vi "Recall aNETka (batch).vi"() -> ()   [LabVIEW 2010]
uses:
  <vilib>/Utility/file.llb/Read From Spreadsheet File (DBL).vi
panel:
  in  "Case Constant\n(See Context Help) 2":bool
  in  "Case Constant\n(See Context Help)":bool
  out "Output Array":sgl[](array[numeric])=[0.04986743, 0.15020862, 0.24986751, 0.34442046, 0.44537312, 0.54999864, 0.6508218, 0.7484142, 0.8519573, 0.94851804] format="%.2f"
  out "New file:":path=path "D:/aNETka/example 2 inputs, 1 output (aNETka).txt"
  out "Waveform Graph":sgl[][](graph)=[[0.04986743], [0.15020862], [0.24986751], [0.34442046], [0.44537312], [0.54999864], [0.6508218], [0.7484142], [0.8519573], [0.94851804]]
  out "aNETka config":i32[](array[numeric])=[2, 5, 1]
  out "Input file:":path=path "D:/aNETka/example 2 inputs, 1 output.txt"
  out "Function":enum16{"Linear", "Sigmoid", "Tangent hyp."}(ring)=enum."Sigmoid"
  out "aNETka config":i32[](array[numeric])=[2, 5, 1] min=0 max=100 step=1
  out "aNETka configuration":cluster{dbl[], dbl[]}[](graph)=[{[2.0, 3.0], [5.5, 3.5]}, {[2.0, 3.0], [4.5, 3.5]}, {[2.0, 3.0], [3.5, 3.5]}, {[2.0, 3.0], [2.5, 3.5]}, {[2.0, 3.0], [1.5, 3.5]}, {[1.0, 2.0], [4.0, 1.5]}, {[1.0, 2.0], [4.0, 2.5]}, {[1.0, 2.0], [4.0, 3.5]}, {[1.0, 2.0], [4.0, 4.5]}, {[1.0, 2.0], [4.0, 5.5]}, {[1.0, 2.0], [3.0, 1.5]}, {[1.0, 2.0], [3.0, 2.5]}, {[1.0, 2.0], [3.0, 3.5]}, {[1.0, 2.0], [3.0, 4.5]}, {[1.0, 2.0], [3.0, 5.5]}]
  # "Inputs"
  # "Outputs"
  # "(Hidden layers)"
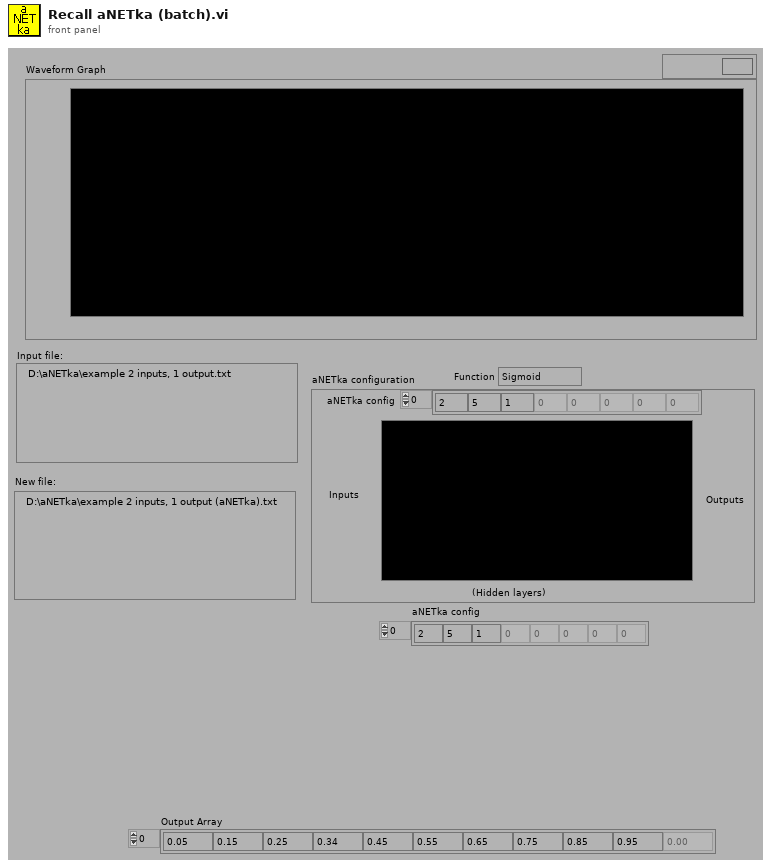
[diagram p1: front panel]
types:
  T1 = enum32{"existing file", "new file", "new or existing file", "existing dir", "new dir", "new or existing dir", "existing file (use LLBs)", "new file (use LLBs)", "new or existing file (use LLBs)", "new or existing file or directory (use LLBs)"}
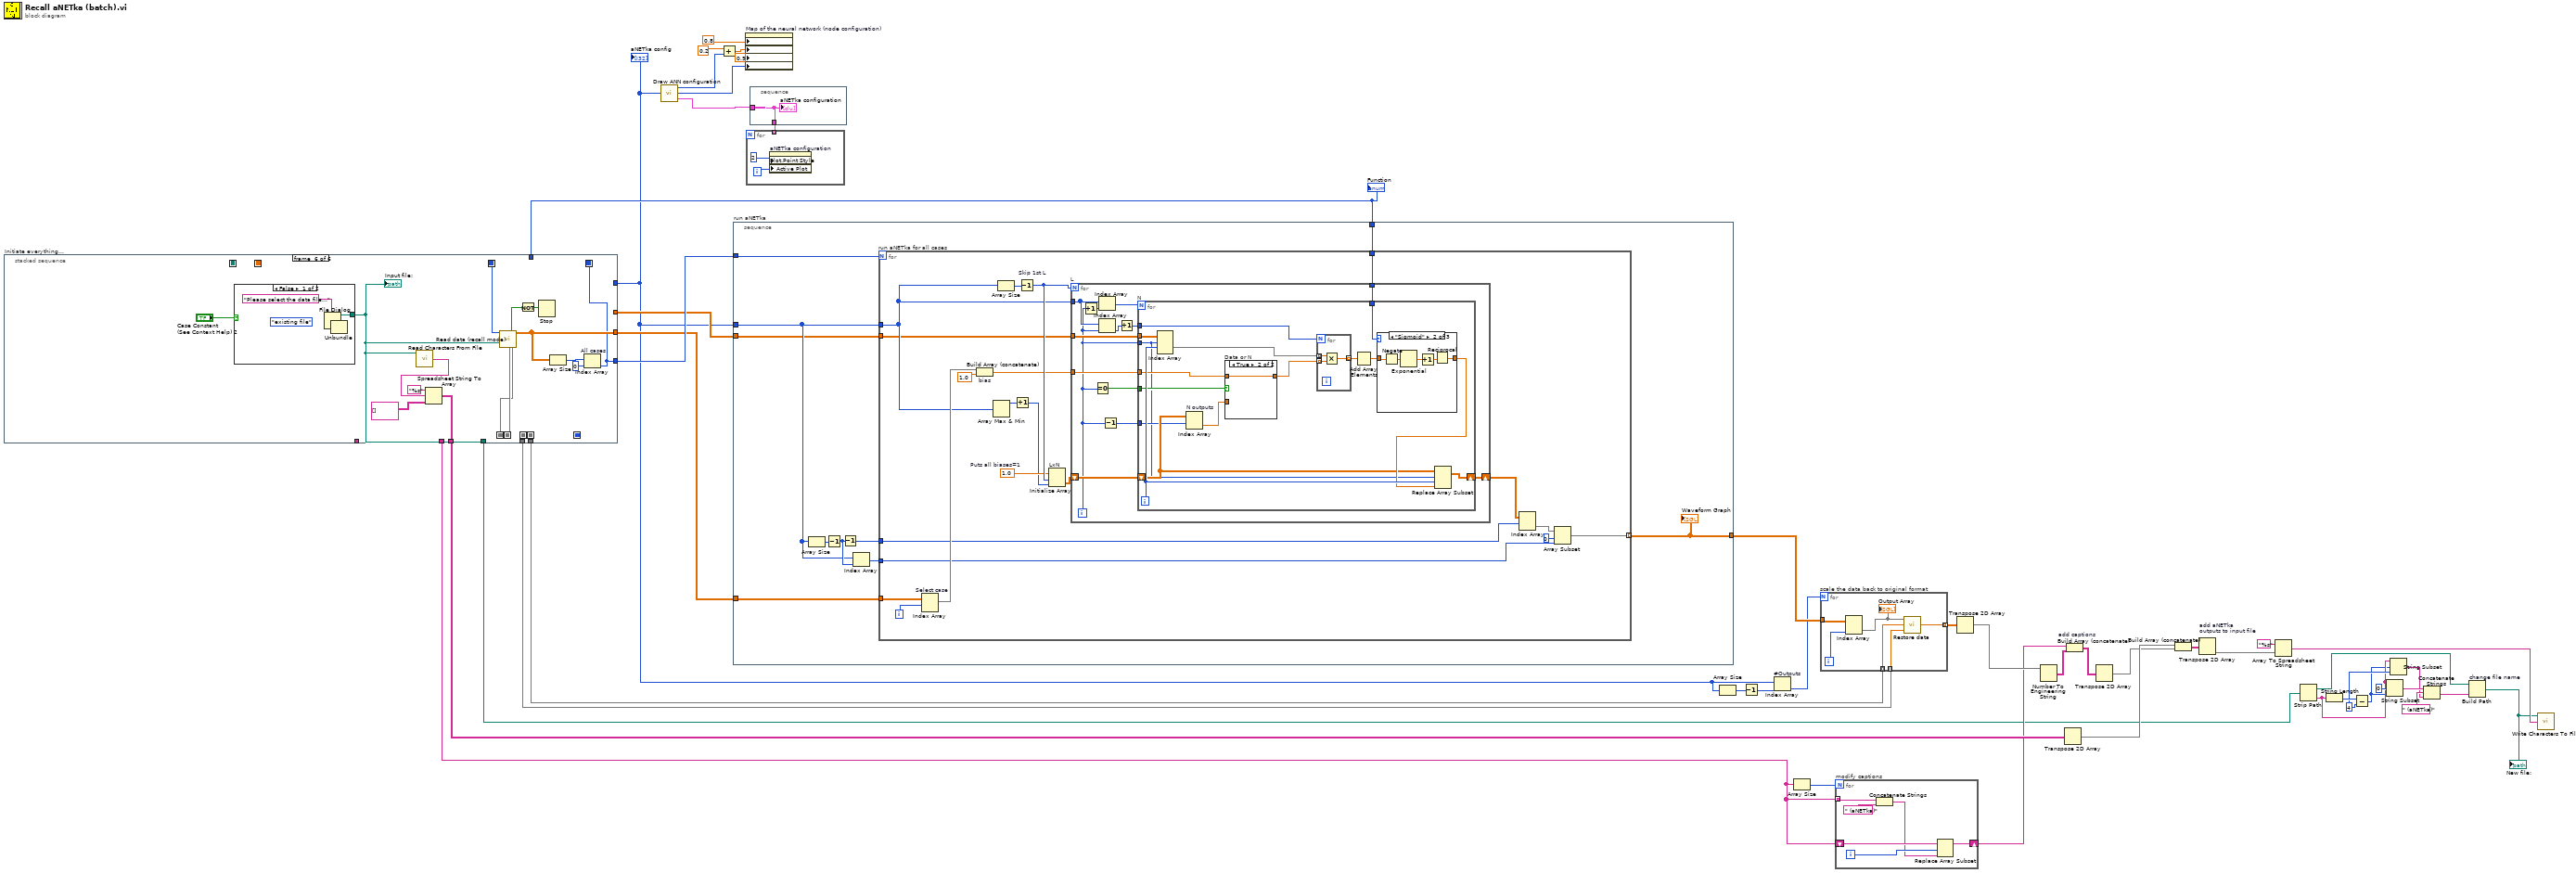
[diagram p0: block diagram]
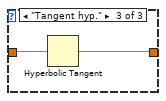
[diagram p3: hidden frame]
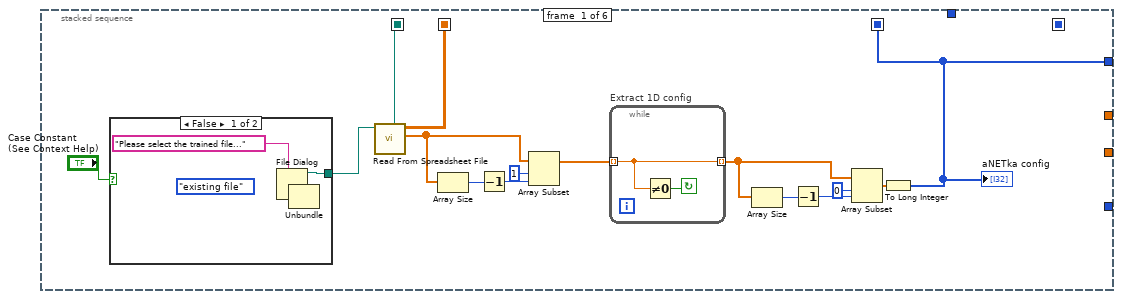
[diagram p5: hidden frame]
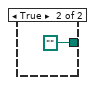
[diagram p6: hidden frame]
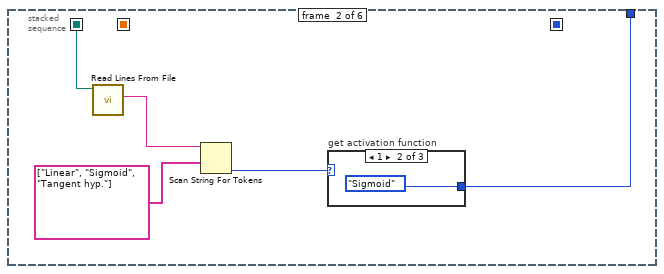
[diagram p7: hidden frame]
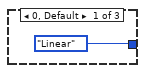
[diagram p8: hidden frame]
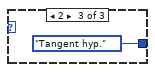
[diagram p9: hidden frame]
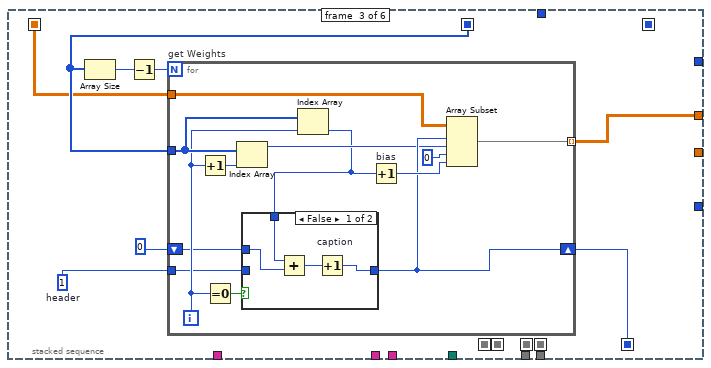
[diagram p10: hidden frame]
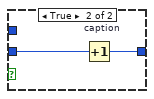
[diagram p11: hidden frame]
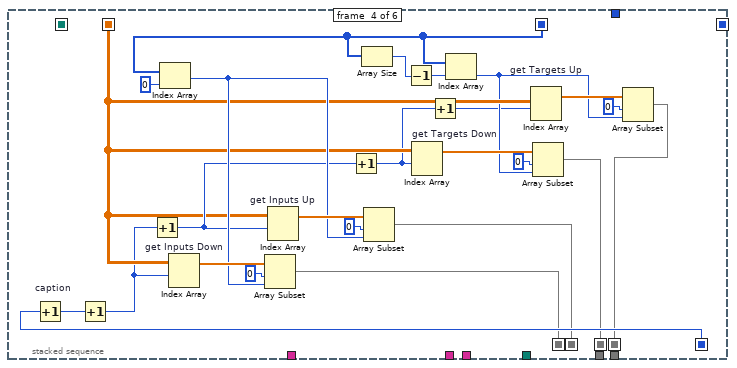
[diagram p12: hidden frame]
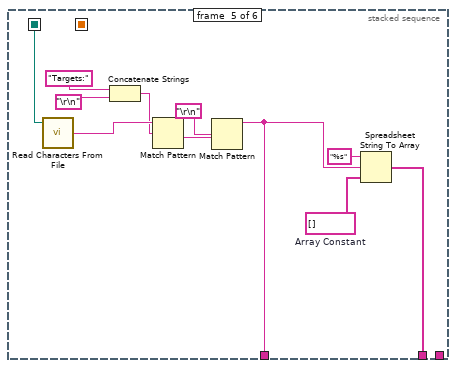
[diagram p13: hidden frame]
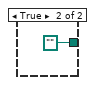
[diagram p14: hidden frame]
diagram:
  w11 = 4 ("y")
  n1 = stacked-sequence "Initiate everything..." {
    seq-local: [w49 _ _ _ _ _] -> [_ _ w80 w115 _ w150]
    seq-local: [_ _ _ _ _ w146] -> [_ _ _ _ _ _]
    seq-local: [w50 _ _ _ _ _] -> [_ _ w79 w110 _ _]
    seq-local: [w48 _ _ _ _ _] -> [_ w71 _ _ w137 _]
    seq-local: [_ _ w75 _ _ _] -> [_ _ _ w126 _ _]
    seq-local: [_ _ _ w105 _ _] -> [_ _ _ _ _ w143]
    seq-local: [_ _ _ w104 _ _] -> [_ _ _ _ _ w144]
    seq-local: [_ _ _ w102 _ _] -> [_ _ _ _ _ _]
    seq-local: [_ _ _ w103 _ _] -> [_ _ _ _ _ _]
    tunnel: [w49 _ _ _ _ _] -> w28
    tunnel: [_ w67 _ _ _ _] -> w37
    tunnel: [_ _ _ _ _ w147] -> w34
    tunnel: [_ _ _ _ _ w146] -> w36
    tunnel: [_ _ _ _ _ w138] -> w2
    tunnel: [_ _ w76 _ _ _] -> w35
    tunnel: [_ _ _ _ w130 _] -> _
    tunnel: [_ _ _ w103 _ _] -> w27
    tunnel: [_ _ _ w102 _ _] -> w26
    tunnel: [_ _ _ _ _ w139] -> w25
    tunnel: [_ _ _ _ w127 _] -> w17
    frame #0 {
      n2 = case shown="False" "Case Constant\n(See Context Help)" {
        tunnel: [w64 path ""] -> w46
        frame False {
          (unwired) T1."existing file" ("select mode (2)")
          n3 = File Dialog(7:"Please select the trained file..." ("prompt")) -> (0:w63:errorcluster, 3:w64:path)  [unwired: 6 in, 2 out]
          n4 = Unbundle(w63) -> ()  [unwired: 3 out]
        }
        frame True {
        }
      }
      n5 = call-poly <vilib>:"Read From Spreadsheet File.vi"("file path (dialog if empty)"=w46) -> ("first row"=w57:dbl[], "all rows"=w50:dbl[][], "new file path (Not A Path if cancelled)"=w48:path)  [unwired: 6 in, 2 out]
      n6 = Array Size(array=w57) -> (size(s)=w59:i32)
      n7 = Decrement(x=w59) -> (x-1=w58:i32)
      n8 = Array Subset(array=w57, index=1 ("Array Index"), length=w58) -> (w56:dbl[])
      n9 = while "Extract 1D config" {
        tunnel: [w61] -> w54 mode=indexing
        tunnel: w56 -> [w61] mode=indexing
        stop <- w62 continue-if-true
        n10 = Not Equal To 0?(x=w61) -> (x != 0?=w62:bool)
      }
      n11 = Array Size(array=w54) -> (size(s)=w55:i32)
      n12 = Decrement(x=w55) -> (x-1=w53:i32)
      n13 = Array Subset(array=w54, index=0 ("Array Index"), length=w53) -> (w51:dbl[])
      n14 = To Long Integer(number=w51) -> (32bit integer=w49:i32[])
      "aNETka config" <- w49
    }
    frame #1 {
      n15 = call <vilib>:"Read Lines From File.vi"("file path (dialog if empty)"=w71) -> ("line string"=w70:string)  [unwired: 5 in, 3 out]
      n16 = Scan String For Tokens(7:string[] ["Linear", "Sigmoid", "Tangent hyp."] ("operators (none)"), 9:w70) -> (0:w68:i32)  [unwired: 4 in, 3 out]
      n17 = case "get activation function" shown="1" w68 {
        tunnel: [enum16{"Linear", "Sigmoid", "Tangent hyp."}."Linear" ("Function 2") enum16{"Linear", "Sigmoid", "Tangent hyp."}."Sigmoid" ("Function 2") enum16{"Linear", "Sigmoid", "Tangent hyp."}."Tangent hyp." ("Function 2")] -> w67
        frame 0, Default {
        }
        frame 1 {
        }
        frame 2 {
        }
      }
    }
    frame #2 {
      w78 = 1  # header
      n18 = Array Size(array=w80) -> (size(s)=w82:i32)
      n19 = Decrement(x=w82) -> (x-1=w81:i32)
      n20 = for "get Weights" {
        N: w81 -> [_]
        tunnel: w80 -> [w94]
        tunnel: w79 -> [w89]
        tunnel: [w88] -> w76 mode=indexing
        tunnel: w78 -> [w87]
        shift-right: [w85] -> w75
        shift-left: 0 -> [w86]
        i -> [w90]
        n21 = Increment(x=w90) -> (x+1=w95:i32)
        n22 = Equal To 0?(x=w90) -> (x = 0?=w91:bool)
        n23 = Index Array(array=w94, index=w95) -> (element=w84:i32)
        n24 = Index Array(array=w94, index=w90) -> (element=w83:i32)
        n25 = case shown="False" w91 {
          tunnel: [w97 w101] -> w85
          tunnel: w87 -> [_ w100]
          tunnel: w83 -> [w99 _]
          tunnel: w86 -> [w96 _]
          frame False {
            n26 = Add(x=w99, y=w96) -> (x+y=w98:i32)
            n27 = Increment "caption"(x=w98) -> (x+1=w97:i32)
          }
          frame True {
            n28 = Increment "caption"(x=w100) -> (x+1=w101:i32)
          }
        }
        n29 = Increment "bias"(x=w83) -> (x+1=w92:i32)
        n30 = Array Subset(array=w89, index (row)=w85, length (row)=w84, index (col)=0 ("Array Index"), length (col)=w92) -> (w88:dbl[][])
      }
    }
    frame #3 {
      n31 = Increment "caption"(x=w126) -> (x+1=w119:i32)
      n32 = Increment(x=w119) -> (x+1=w106:i32)
      n33 = Increment(x=w106) -> (x+1=w116:i32)
      n34 = Index Array(array=w115, index=0 ("Index")) -> (element=w120:i32)
      n35 = Index Array "get Inputs Down"(array=w110, index (row)=w106) -> (element=w124:dbl[])  [unwired: 1 in]
      n36 = Array Subset(array=w124, index=0 ("Array Index"), length=w120) -> (w105:dbl[])
      n37 = Index Array "get Inputs Up"(array=w110, index (row)=w116) -> (element=w121:dbl[])  [unwired: 1 in]
      n38 = Increment(x=w116) -> (x+1=w108:i32)
      n39 = Array Size(array=w115) -> (size(s)=w114:i32)
      n40 = Array Subset(array=w121, index=0 ("Array Index"), length=w120) -> (w104:dbl[])
      n41 = Decrement(x=w114) -> (x-1=w113:i32)
      n42 = Index Array "get Targets Down"(array=w110, index (row)=w108) -> (element=w117:dbl[])  [unwired: 1 in]
      n43 = Increment(x=w108) -> (x+1=w107:i32)
      n44 = Index Array(array=w115, index=w113) -> (element=w109:i32)
      n45 = Index Array "get Targets Up"(array=w110, index (row)=w107) -> (element=w112:dbl[])  [unwired: 1 in]
      n46 = Array Subset(array=w117, index=0 ("Array Index"), length=w109) -> (w102:dbl[])
      n47 = Array Subset(array=w112, index=0 ("Array Index"), length=w109) -> (w103:dbl[])
    }
    frame #4 {
      w128 = string[] []  # Array Constant
      n48 = call <vilib>:"Read Characters From File.vi"("file path (dialog if empty)"=w137) -> ("character string"=w136:string)  [unwired: 5 in, 3 out]
      n49 = Concatenate Strings("Targets:" ("regular expression"), "\r\n") -> (w133:string)
      n50 = Match Pattern(string=w136, regular expression=w133) -> (after substring=w131:string)  [unwired: 1 in, 3 out]
      n51 = Match Pattern(string=w131, regular expression="\r\n") -> (before substring=w130:string)  [unwired: 1 in, 3 out]
      n52 = Spreadsheet String To Array(format string="%s", spreadsheet string=w130, array type (2D Dbl)=w128) -> (array=w127:string[])  [unwired: 1 in]
    }
    frame #5 {
      n53 = case shown="False" "Case Constant\n(See Context Help) 2" {
        tunnel: [w154 path ""] -> w138
        frame False {
          (unwired) T1."existing file" ("select mode (2)")
          n54 = File Dialog(7:"Please select the data file..." ("prompt")) -> (0:w153:errorcluster, 3:w154:path)  [unwired: 6 in, 2 out]
          n55 = Unbundle(w153) -> ()  [unwired: 3 out]
        }
        frame True {
        }
      }
      "Input file:" <- w138
      n56 = call <vilib>:"Read Characters From File.vi"("file path (dialog if empty)"=w138) -> ("character string"=w142:string)  [unwired: 5 in, 3 out]
      n57 = Spreadsheet String To Array(format string="%s", spreadsheet string=w142, array type (2D Dbl)=string[][] []) -> (array=w139:string[][])  [unwired: 1 in]
      n58 = call "Read data (recall mode).vi"("aNETka config"=w150, "Data file path"=w138, "Up Inputs"=w144, "Down Inputs"=w143) -> ("Continue? (T=yes)"=w152:bool, "Scaled inputs"=w147:sgl[][])  [unwired: 12 in, 2 out]
      n59 = Not(x=w152) -> (.not. x?=w151:bool)
      n60 = Stop(stop? (T)=w151) -> ()
      n61 = Array Size(array=w147) -> (size(s)=w148:i32[])
      n62 = Index Array "All cases"(array=w148, index=0 ("Index")) -> (element=w146:i32)
    }
  }
  "aNETka config" <- w28
  "Function" <- w37
  n63 = call "Draw ANN configuration.vi"("Array"=w28) -> ("Xmax"=w45:i8, "Ymax"=w42:i16, "Map of the neural network (node configuration)"=w39:cluster{dbl[], dbl[]}[])
  n64 = Add(x=0.2, y=w45) -> (x+y=w43:dbl)
  n65 = stacked-sequence "run aNETka" {
    tunnel: w34 -> [w166]
    tunnel: w37 -> [w165]
    tunnel: w36 -> [w164]
    tunnel: w28 -> [w159]
    tunnel: w35 -> [w158]
    tunnel: [w157] -> w32
    frame #0 {
      n66 = Array Size(array=w159) -> (size(s)=w162:i32)
      n67 = Decrement(x=w162) -> (x-1=w163:i32)
      n68 = Decrement(x=w163) -> (x-1=w161:i32)
      n69 = Index Array(array=w159, index=w163) -> (element=w160:i32)
      n70 = for "run aNETka for all cases" {
        N: w164 -> [_]
        tunnel: w159 -> [w172]
        tunnel: w165 -> [w183]
        tunnel: w166 -> [w186]
        tunnel: w161 -> [w171]
        tunnel: w160 -> [w170]
        tunnel: w158 -> [w169]
        tunnel: [w167] -> w157 mode=indexing
        i -> [w168]
        w178 = sgl 1.0  # Puts all biases=1
        n71 = Index Array "Select case"(array=w186, index (row)=w168) -> (element=w182:sgl[])  [unwired: 1 in]
        n72 = Build Array (concatenate) "bias"(w182, sgl 1.0 ("Input Element")) -> (w173:sgl[])
        n73 = Array Max & Min(array=w172) -> (max value=w177:i32)  [unwired: 3 out]
        n74 = Array Size(array=w172) -> (size(s)=w179:i32)
        n75 = Increment(x=w177) -> (x+1=w175:i32)
        n76 = Decrement "Skip 1st L"(x=w179) -> (x-1=w180:i32)
        n77 = Initialize Array "LxN"(w178, w180, w175) -> (w176:sgl[][])
        n78 = for "L" {
          N: w180 -> [_]
          shift-right: [w199] -> w181
          shift-left: w176 -> [w189]
          tunnel: w172 -> [w193]
          tunnel: w173 -> [w195]
          tunnel: w183 -> [w194]
          tunnel: w169 -> [w191]
          i -> [w187]
          n79 = Increment(x=w187) -> (x+1=w198:i32)
          n80 = Equal To 0?(x=w187) -> (x = 0?=w196:bool)
          n81 = Index Array(array=w193, index=w187) -> (element=w192:i32)
          n82 = Index Array(array=w193, index=w198) -> (element=w197:i32)
          n83 = Decrement(x=w187) -> (x-1=w188:i32)
          n84 = Increment(x=w192) -> (x+1=w190:i32)
          n85 = for "N" {
            N: w197 -> [_]
            shift-right: [w215] -> w199
            shift-left: w189 -> [w203]
            tunnel: w187 -> [w201]
            tunnel: w196 -> [w213]
            tunnel: w195 -> [w211]
            tunnel: w194 -> [w212]
            tunnel: w190 -> [w205]
            tunnel: w191 -> [w208]
            tunnel: w188 -> [w202]
            i -> [w214]
            n86 = Index Array(array=w208, index (dim 0)=w201, index (dim 1)=w214) -> (element=w207:dbl[])  [unwired: 1 in]
            n87 = Index Array "N outputs"(array=w203, index (row)=w202) -> (element=w206:sgl[])  [unwired: 1 in]
            n88 = case "Data or N" shown="True" w213 {
              tunnel: w206 -> [w227 _]
              tunnel: w211 -> [_ w228]
              tunnel: [w227 w228] -> w200
              frame False {
              }
              frame True {
              }
            }
            n89 = for {
              N: w205 -> [_]
              tunnel: [w218] -> w210 mode=indexing
              tunnel: w207 -> [w217] mode=indexing
              tunnel: w200 -> [w216] mode=indexing
              n90 = Multiply(x=w217, y=w216) -> (x*y=w218:dbl)
            }
            n91 = Add Array Elements(numeric array=w210) -> (sum=w209:dbl)
            n92 = case shown="\"Sigmoid\"" w212 {
              tunnel: w209 -> [w219 w221 w226]
              tunnel: [w219 w220 w225] -> w204
              frame "Linear", Default {
              }
              frame "Sigmoid" {
                n93 = Negate(x=w221) -> (-x=w224:dbl)
                n94 = Exponential(1:w224) -> (0:w223:dbl)
                n95 = Increment(x=w223) -> (x+1=w222:dbl)
                n96 = Reciprocal(x=w222) -> (1/x=w220:dbl)
              }
              frame "Tangent hyp." {
                n97 = Hyperbolic Tangent(1:w226) -> (0:w225:dbl)
              }
            }
            n98 = Replace Array Subset(array=w203, new element=w204, index (row)=w201, index (col)=w214) -> (w215:sgl[][])
          }
        }
        n99 = Index Array(array=w181, index (row)=w171) -> (element=w184:sgl[])  [unwired: 1 in]
        n100 = Array Subset(array=w184, index=0 ("Array Index"), length=w170) -> (w167:sgl[])
      }
      "Waveform Graph" <- w157
    }
  }
  n101 = property on="Map of the neural network (node configuration)" class="XYGraph (strict)"("X Scale.Range:Minimum"=0.8, "X Scale.Range:Maximum"=w43, "Y Scale.Range:Minimum"=0.9, "Y Scale.Range:Maximum"=w42) -> ()  [unwired: 2 in, 2 out]
  n102 = stacked-sequence {
    tunnel: w39 -> [w229]
    tunnel: [w229] -> w38
    frame #0 {
      "aNETka configuration" <- w229
    }
  }
  n103 = for {
    tunnel: w38 -> [_] mode=indexing
    i -> [w230]
    n104 = property on="aNETka configuration" class="XYGraph (strict)"("Plot.Point Style"=u8 2 ("Write Attribute"), "Active Plot"=w230) -> ()  [unwired: 2 in, 2 out]
  }
  n105 = Array Size(array=w28) -> (size(s)=w31:i32)
  n106 = Decrement(x=w31) -> (x-1=w30:i32)
  n107 = Index Array "#Outputs"(array=w28, index=w30) -> (element=w29:i32)
  n108 = Array Size(array=w17) -> (size(s)=w18:i32)
  n109 = for "scale the data back to original format" {
    N: w29 -> [_]
    tunnel: w32 -> [w236]
    tunnel: [w235] -> w33 mode=indexing
    tunnel: w27 -> [w233] mode=indexing
    tunnel: w26 -> [w232] mode=indexing
    i -> [w237]
    n110 = Index Array(array=w236, index (col)=w237) -> (element=w234:sgl[])  [unwired: 1 in]
    "Output Array" <- w234
    n111 = call "Restore data.vi"("Offset down"=w232, "Offset up"=w233, "Scaled data"=w234) -> ("Restored data"=w235:sgl[])
  }
  n112 = for "modify captions" {
    N: w18 -> [_]
    tunnel: w17 -> [w243] mode=indexing
    shift-right: [w238] -> w16
    shift-left: w17 -> [w240]
    i -> [w241]
    n113 = Concatenate Strings(w243, " (aNETka)") -> (w239:string)
    n114 = Replace Array Subset(array=w240, new element=w239, index=w241) -> (w238:string[])
  }
  n115 = Transpose 2D Array(2D array=w33) -> (transposed array=w24:sgl[][])
  n116 = Number To Engineering String(4:w24) -> (0:w20:string[][])  [unwired: 3 in]
  n117 = Transpose 2D Array(2D array=w25) -> (transposed array=w22:string[][])
  n118 = Build Array (concatenate) "add captions"(w16, w20) -> (w19:string[][])
  n119 = Transpose 2D Array(2D array=w19) -> (transposed array=w21:string[][])
  n120 = Build Array (concatenate)(w22, w21) -> (w23:string[][])
  n121 = Transpose 2D Array "add aNETka\noutputs to input file"(2D array=w23) -> (transposed array=w5:string[][])
  n122 = Array To Spreadsheet String(array=w5, 3:"%s" ("format string")) -> (spreadsheet string=w3:string)  [unwired: 1 in]
  n123 = Strip Path(path=w2) -> (stripped path=w7:path, name=w10:string)
  n124 = String Length(string=w10) -> (length=w15:i32)
  n125 = Subtract(x=w15, y=w11) -> (x-y=w6:i32)
  n126 = String Subset(string=w10, offset (0)=0, length (rest)=w6) -> (substring=w13:string)
  n127 = String Subset(string=w10, offset (0)=w6, length (rest)=w11) -> (substring=w9:string)
  n128 = Concatenate Strings(w13, " (aNETka)", w9) -> (w8:string)
  n129 = Build Path "change file name"(base path=w7, name or relative path=w8) -> (appended path=w1:path)
  "New file:" <- w1
  n130 = call <vilib>:"Write Characters To File.vi"("character string"=w3, "file path (dialog if empty)"=w1) -> ()  [unwired: 3 in, 1 out]
